vi "Process.vi"(8 "error in":errorcluster, 9 "Logging":cluster{"Enabled?":bool, "Log Path":path}, 10 "watchdogID":u64, 11 "Pound":refnum<class "Pound.lvclass">) -> (0 "error out":errorcluster, 1 "ExpirationType":T1, 2 "Expired Process":string)   [LabVIEW 2017, in "WatchdogProcess.lvlib"]
doc: "Creates a watchdog when the process starts running. Each time the process While Loop iterates, this package resets the timer. If the timer reaches zero, the Watchdog process restarts the device."
uses:
  <vilib>/addons/WatchdogProcess/WatchdogProcess.lvlib
  <vilib>/NI/Software Watchdog/Pound/ExpirationType.ctl
  <vilib>/NI/Software Watchdog/Pound/Pound.lvclass
  <vilib>/nisyscfg/nisyscfg.lvlib
  <vilib>/nisyscfg/Close (System).vi
  <vilib>/addons/SystemInfoProcess/SystemInfoProcess.lvlib
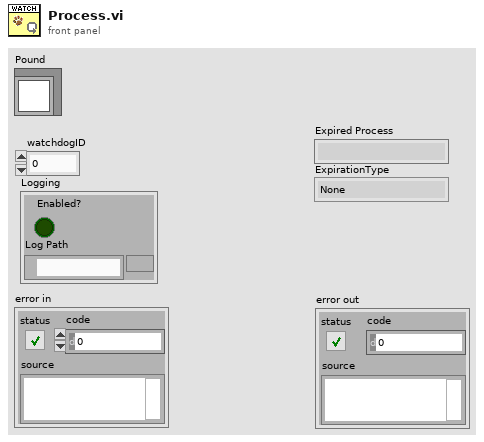
[diagram p1: front panel]
types:
  T1 = typedef "Pound.lvclass/ExpirationType.ctl" = enum16{"None", "Execution", "Shutdown"}
  T2 = typedef "PointValueMap.lvlib/PointMap.ctl" = refnum<data-value>
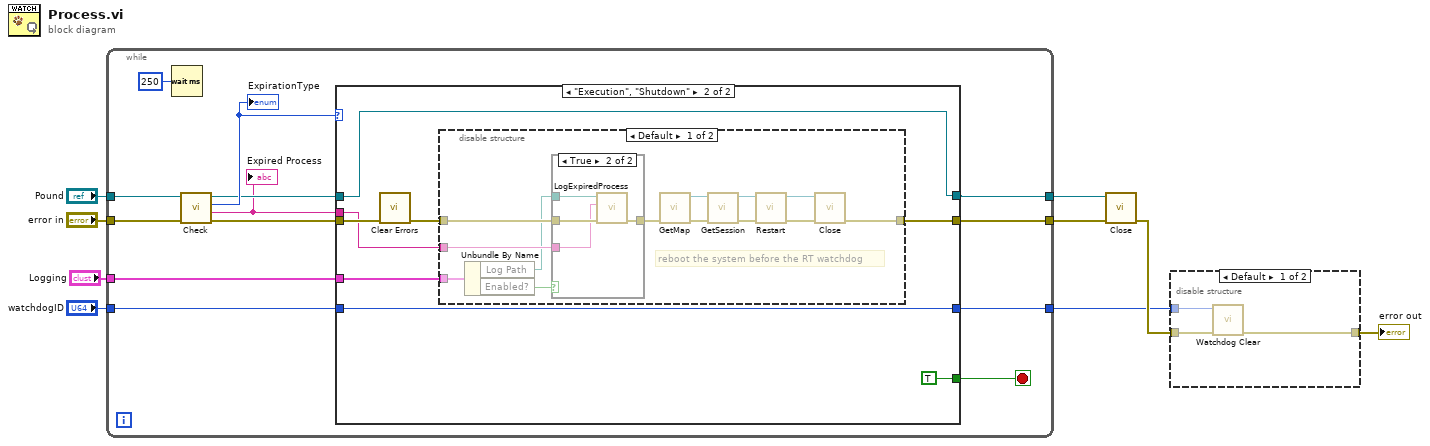
[diagram p0: block diagram]
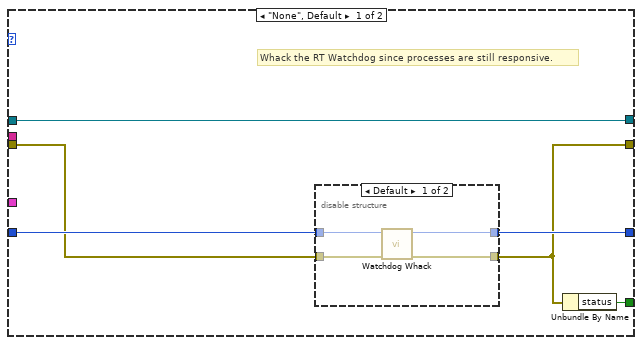
[diagram p3: hidden frame]
diagram:
  n1 = while {
    tunnel: "Pound" -> [w22]
    tunnel: [w13] -> w5
    tunnel: "error in" -> [w21]
    tunnel: [w15] -> w6
    tunnel: "watchdogID" -> [w17]
    tunnel: [w16] -> w3
    tunnel: "Logging" -> [w10]
    stop <- w12 stop-if-true
    n2 = Wait (ms)(milliseconds to wait=u32 250) -> ()  [unwired: 1 out]
    n3 = call <vilib>:"Check.vi"("error in (no error)"=w21, "Pound"=w22) -> ("error out"=w18:errorcluster, "Watchdog Name"=w11:string, "ExpirationType"=w19:T1, "Pound"=w14:refnum<class "Pound.lvclass">)  [unwired: 6 in]
    "Expired Process" <- w11
    "ExpirationType" <- w19
    n4 = case shown="\"Execution\", \"Shutdown\"" w19 {
      tunnel: w18 -> [w27 w38]
      tunnel: [w24 w40] -> w15
      tunnel: w17 -> [w28 w42]
      tunnel: [w26 w42] -> w16
      tunnel: [w25 TRUE] -> w12
      tunnel: w14 -> [w23 w39]
      tunnel: [w23 w39] -> w13
      tunnel: w11 -> [_ w36]
      tunnel: w10 -> [_ w35]
      frame "None", Default {
        # "Whack the RT Watchdog since processes are still responsive."
        n5 = disable-structure shown="Default" {
          disable-tunnel: w28 -> [w32 w34]
          disable-tunnel: w27 -> [w31 w33]
          disable-tunnel: [w30 w34] -> w26
          disable-tunnel: [w29 w33] -> w24
          frame condition #0 {
            n6 = call <vilib>:"Watchdog Whack.vi"("error in (no error)"=w31, "watchdogID in"=w32) -> ("error out"=w29:errorcluster, "watchdogID out"=w30:u64)  [unwired: 3 in, 1 out]
          }
          frame condition #1 (active) {
          }
        }
        n7 = Unbundle By Name(w24) -> ("status"=w25:bool)
      }
      frame "Execution", "Shutdown" {
        n8 = call <vilib>:"Clear Errors.vi"("error in (no error)"=w38) -> ("error out"=w37:errorcluster)  [unwired: 5 in, 1 out]
        n9 = disable-structure shown="Default" {
          disable-tunnel: [w55 w61] -> w40
          disable-tunnel: w37 -> [w48 w61]
          disable-tunnel: w36 -> [w46 _]
          disable-tunnel: w35 -> [w45 _]
          frame condition #0 {
            # "reboot the system before the RT watchdog"
            n10 = Unbundle By Name(w45) -> ("Log Path"=w43:path, "Enabled?"=w44:bool)
            n11 = case shown="True" w44 {
              tunnel: w48 -> [w56 w60]
              tunnel: [w56 w59] -> w47
              tunnel: w46 -> [_ w58]
              tunnel: w43 -> [_ w57]
              frame False {
              }
              frame True {
                n12 = call <vilib>:"LogExpiredProcess.vi"("error in"=w60, "Expired Process"=w58, "Path"=w57) -> ("error out"=w59:errorcluster)  [unwired: 8 in]
              }
            }
            n13 = call <vilib>:"GetMap.vi"("error in (no error)"=w47) -> ("error out"=w51:errorcluster, "SystemInfoMap"=w52:T2)  [unwired: 9 in]
            n14 = call <vilib>:"GetSession.vi"("error in (no error)"=w51, "map"=w52) -> ("error out"=w50:errorcluster, "session"=w49:refnum<k21>)  [unwired: 8 in]
            n15 = call <vilib>:"Restart.vi"("error in (no error)"=w50, "Session in"=w49) -> ("error out"=w54:errorcluster, "Session out"=w53:refnum<k21>)  [unwired: 7 in, 1 out]
            n16 = call-poly <vilib>:"Close.vi"("error in (no error)"=w54, "Session in"=w53) -> ("error out"=w55:errorcluster)  [unwired: 9 in]
          }
          frame condition #1 (active) {
          }
        }
      }
    }
  }
  n17 = call <vilib>:"Close.vi"("error in (no error)"=w6, "Pound"=w5) -> ("error out"=w4:errorcluster)  [unwired: 9 in]
  n18 = disable-structure shown="Default" {
    disable-tunnel: w4 -> [w64 w65]
    disable-tunnel: w3 -> [w63 _]
    disable-tunnel: [w62 w65] -> w2
    frame condition #0 {
      n19 = call <vilib>:"Watchdog Clear.vi"("error in (no error)"=w64, "watchdogID in"=w63) -> ("error out"=w62:errorcluster)  [unwired: 5 in]
    }
    frame condition #1 (active) {
    }
  }
  "error out" <- w2
